vi "processamento_dos_dados_medios_de_calibracao.vi"() -> ()   [LabVIEW 2011]
uses:
  <vilib>/Analysis/NI_AALBase.lvlib
  <vilib>/Analysis/baseanly.llb/Mean (DBL).vi
panel:
  out "Desvio Padrão do Erro Absoluto (N)":dbl format="%0.2f"
  out "Média do Erro Absoluto (N)":dbl format="%0.2f"
  out "Erro Absoluto da Calibração (N)":dbl[](array[numeric])
  out "Desvio Padrão do Erro Relativo":dbl format="%0.2f"
  out "Média do Erro Relativo":dbl format="%0.2f"
  out "Erro Relativo da Calibração":dbl[](array[numeric])
  out "Dados carregados":dbl[](graph)
  out "XY Graph":cluster{"Y":dbl[], "Y":dbl[]}[](graph)
  out "Força aplicada (N)":dbl[](array[numeric])
  out "Força calculada (N)":dbl[](array[numeric])
  # "PROGRAMA PARA O PROCESSAMENTO DOS DADOS \nDO PROCEDIMENTO DE CALIBRAÇÃO"
  # "Desenvolvido por Eloi Antonio Triaca"
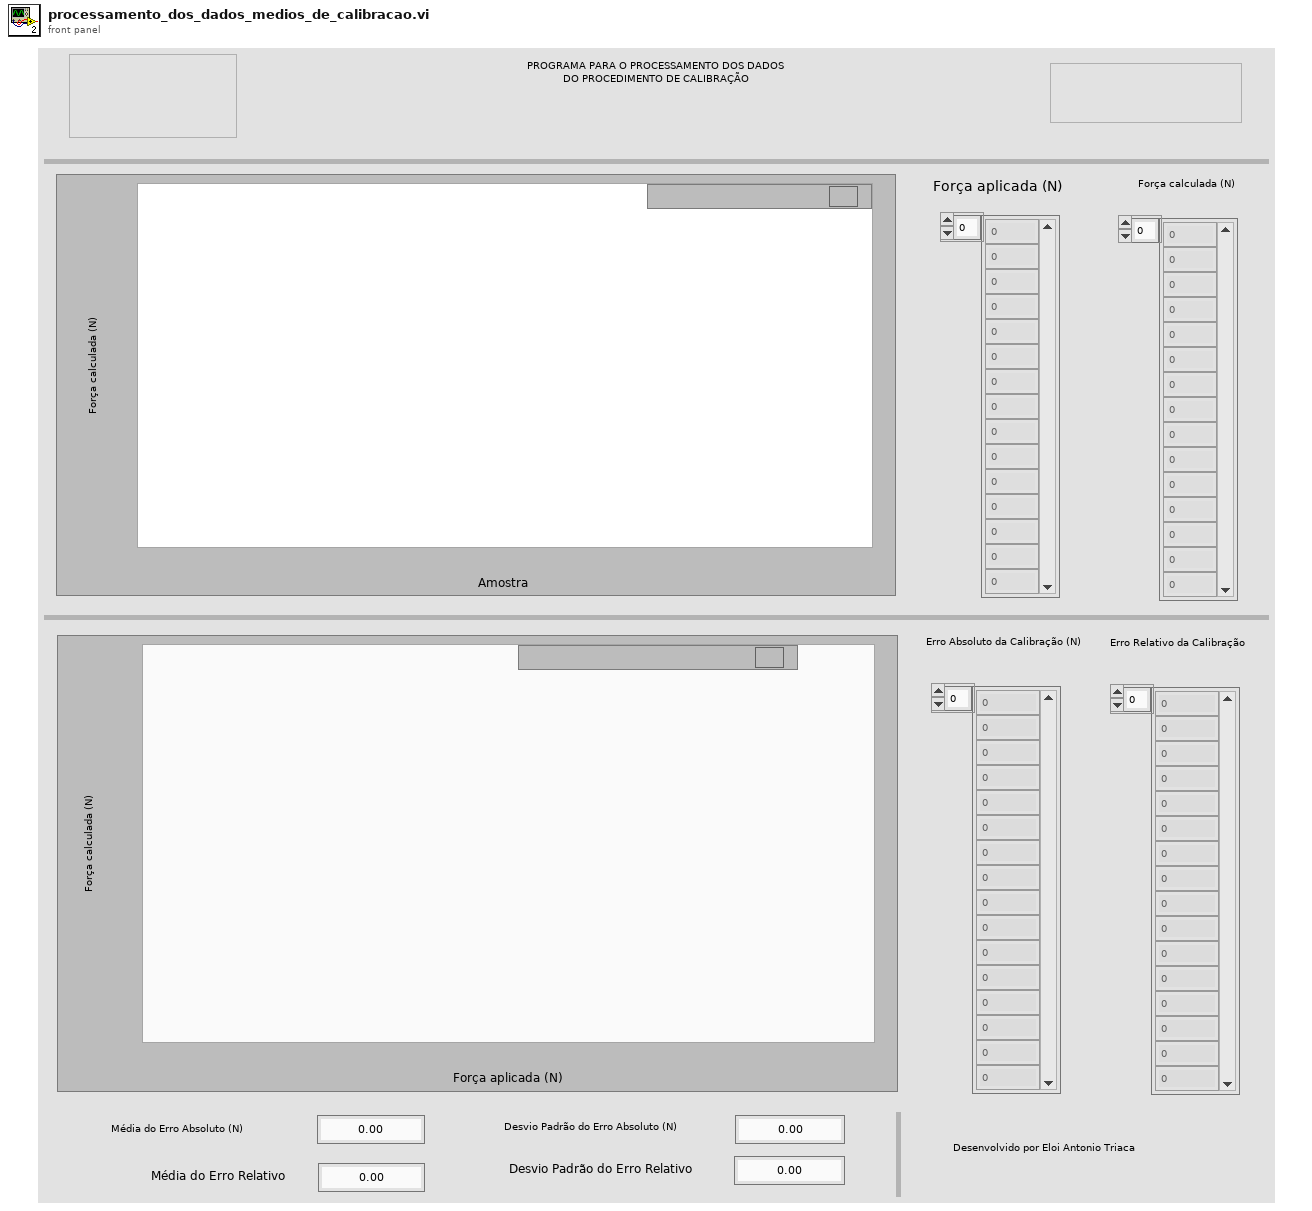
[diagram p1: front panel]
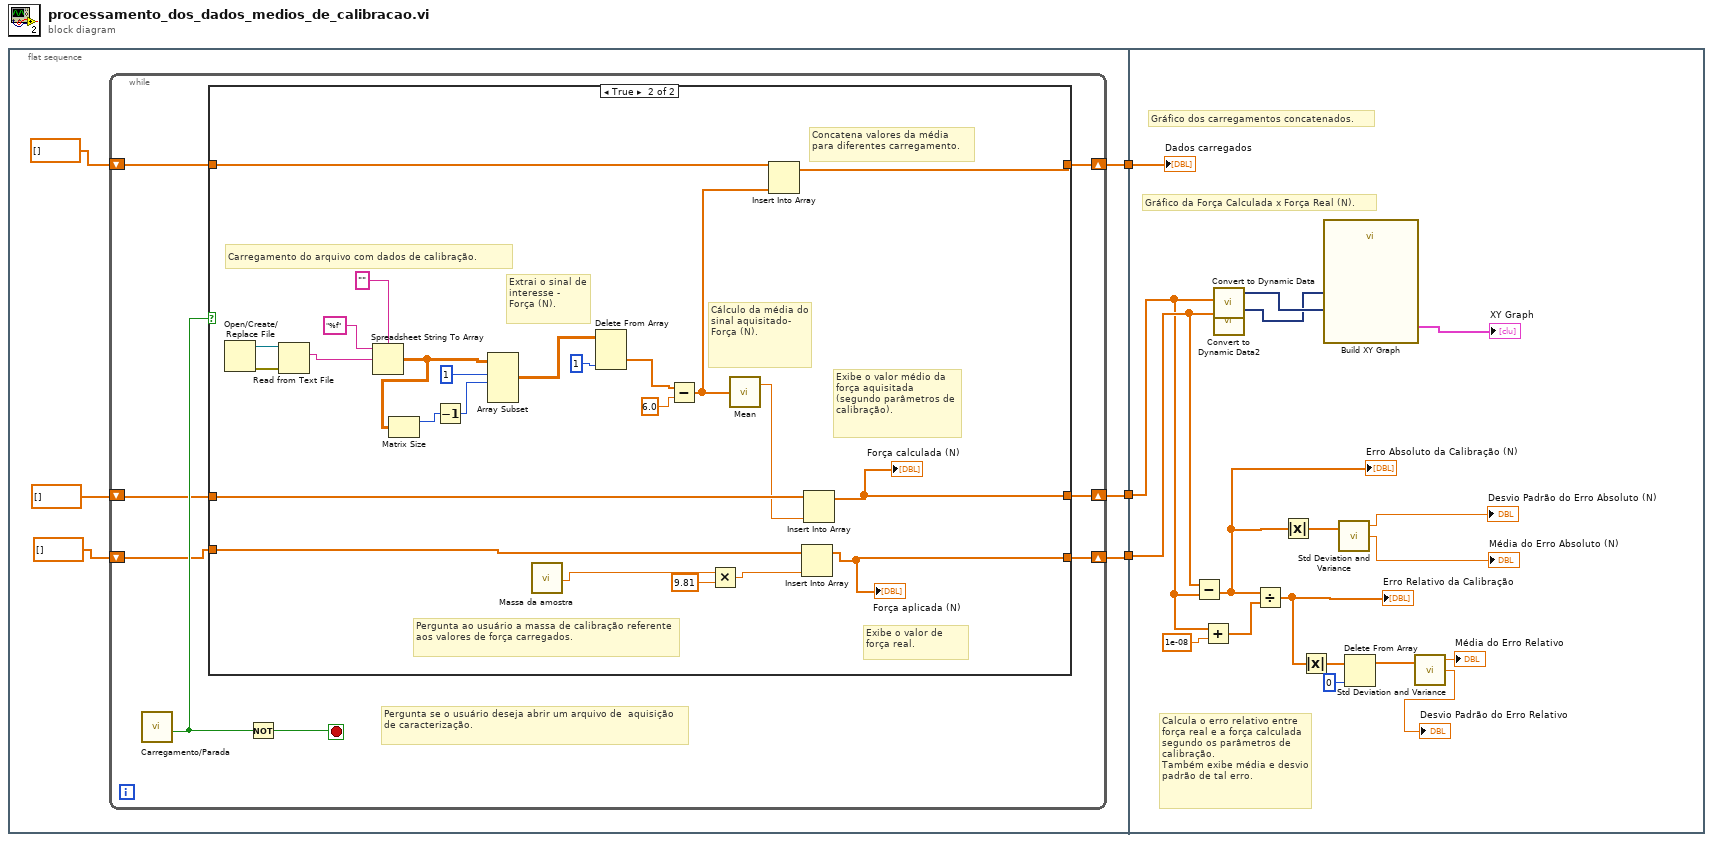
[diagram p0: block diagram]
diagram:
  n1 = flat-sequence {
    tunnel: [w8] -> w3
    tunnel: [w6] -> w2
    tunnel: [w4] -> w1
    tunnel: w3 -> [w61]
    tunnel: w2 -> [w52]
    tunnel: w1 -> [w54]
    frame #0 {
      n2 = while {
        shift-right: [w14] -> w8
        shift-left: dbl[] [] ("array") -> [w15]
        shift-right: [w12] -> w6
        shift-left: dbl[] [] ("array") -> [w13]
        shift-right: [w10] -> w4
        shift-left: dbl[] [] ("array") -> [w11]
        stop <- w17 stop-if-true
        # "Pergunta se o usuário deseja abrir um arquivo de  aquisição de caracterização."
        n3 = call "Carregamento/Parada"() -> ("Carregar"=w16:bool)  [unwired: 18 in, 1 out]
        n4 = case shown="True" w16 {
          tunnel: [w20 w40] -> w14
          tunnel: w15 -> [w20 w39]
          tunnel: w13 -> [w19 w38]
          tunnel: [w19 w34] -> w12
          tunnel: w11 -> [w18 w37]
          tunnel: [w18 w35] -> w10
          frame False {
          }
          frame True {
            # "Concatena valores da média para diferentes carregamento."
            # "Exibe o valor de força real."
            # "Exibe o valor médio da força aquisitada (segundo parâmetros de calibração)."
            # "Cálculo da média do sinal aquisitado-  Força (N)."
            # "Carregamento do arquivo com dados de calibração."
            # "Pergunta ao usuário a massa de calibração referente aos valores de força carregados."
            # "Extrai o sinal de interesse - Força (N)."
            n5 = Open/Create/Replace File() -> (refnum out=w44:refnum<file>, error out=w42:errorcluster)  [unwired: 6 in, 1 out]
            n6 = Read from Text File(file (use dialog)=w44, error in=w42) -> (text=w41:string)  [unwired: 2 in, 3 out]
            n7 = Spreadsheet String To Array(delimiter (Tab)="", format string="%f", spreadsheet string=w41) -> (array=w28:dbl[][])  [unwired: 1 in]
            n8 = Matrix Size(0:w28) -> (1:w30:i32)  [unwired: 1 out]
            n9 = Decrement(x=w30) -> (x-1=w29:i32)
            n10 = Array Subset(array=w28, index (row)=1 ("row 1"), length (row)=w29) -> (w31:dbl[][])  [unwired: 2 in]
            n11 = call "Massa da amostra"() -> ("Massa"=w27:dbl)  [unwired: 17 in, 2 out]
            n12 = Delete From Array(array=w31, index (col)=1 ("disabled index (col)")) -> (deleted portion=w23:dbl[])  [unwired: 2 in, 1 out]
            n13 = Subtract(x=w23, y=6.0) -> (x-y=w21:dbl[])
            n14 = Multiply(x=w27, y=9.81) -> (x*y=w25:dbl)
            n15 = call-poly <vilib>:"Mean.vi"("X"=w21) -> ("mean"=w36:dbl)  [unwired: 1 out]
            n16 = Insert Into Array(array=w39, new element=w21) -> (w40:dbl[])  [unwired: 1 in]
            n17 = Insert Into Array(array=w37, new element=w25) -> (w35:dbl[])  [unwired: 1 in]
            "Força aplicada (N)" <- w35
            n18 = Insert Into Array(array=w38, new element=w36) -> (w34:dbl[])  [unwired: 1 in]
            "Força calculada (N)" <- w34
          }
        }
        n19 = Not(x=w16) -> (.not. x?=w17:bool)
      }
    }
    frame #1 {
      # "Calcula o erro relativo entre força real e a força calculada segundo os parâmetros de calibração.\nTambém exibe média e desvio padrão de tal erro."
      # "Gráfico da Força Calculada x Força Real (N)."
      # "Gráfico dos carregamentos concatenados."
      n20 = Subtract(x=w54, y=w52) -> (x-y=w49:dbl[])
      "Erro Absoluto da Calibração (N)" <- w49
      n21 = Add(x=w52, y=1e-08) -> (x+y=w51:dbl[])
      n22 = call "Convert to Dynamic Data"("Array"=w54) -> ("Dynamic Data Type"=w56:dynamicdata)  [unwired: 3 in]
      n23 = call "Convert to Dynamic Data2"("Array"=w52) -> ("Dynamic Data Type"=w55:dynamicdata)  [unwired: 3 in]
      n24 = Divide(x=w49, y=w51) -> (x/y=w48:dbl[])
      "Erro Relativo da Calibração" <- w48
      n25 = Absolute Value(x=w49) -> (abs(x)=w50:dbl[])
      n26 = Absolute Value(x=w48) -> (abs(x)=w47:dbl[])
      n27 = call "Build XY Graph"("Y Input"=w56, "X Input"=w55) -> ("XY Graph"=→"XY Graph":cluster{"Y":dbl[], "Y":dbl[]}[])  [unwired: 3 in, 6 out]
      n28 = call <vilib>:"Std Deviation and Variance.vi"("X"=w50) -> ("mean"=→"Desvio Padrão do Erro Absoluto (N)":dbl, "standard deviation"=→"Média do Erro Absoluto (N)":dbl)  [unwired: 1 in, 1 out]
      n29 = Delete From Array(array=w47, index=0) -> (array with subset deleted=w45:dbl[])  [unwired: 1 in, 1 out]
      n30 = call <vilib>:"Std Deviation and Variance.vi"("X"=w45) -> ("mean"=→"Média do Erro Relativo":dbl, "standard deviation"=→"Desvio Padrão do Erro Relativo":dbl)  [unwired: 1 in, 1 out]
      "Dados carregados" <- w61
    }
  }
